vi "Get SQL formatted value.vi"(8 "error in (no error)":errorcluster, 11 "Column in":refnum<class "Ctrl Refnum Column.lvclass">) -> (0 "error out":errorcluster, 2 "Formatted Value":string, 3 "Column out":refnum<class "Ctrl Refnum Column.lvclass">)   [LabVIEW 2020, in "Basic Fields.lvlib" / "Ctrl Refnum Column.lvclass"]
uses:
  Ctrl Refnum Column.lvclass
  Ctrl Refnum Column.lvclass/Ctrl Refnum Column.ctl
  Basic Columns/Basic Columns/Column Class/Column Parent.lvclass
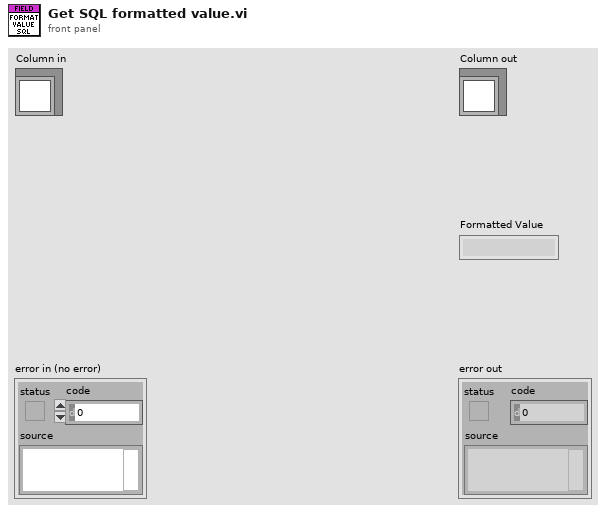
[diagram p1: front panel]
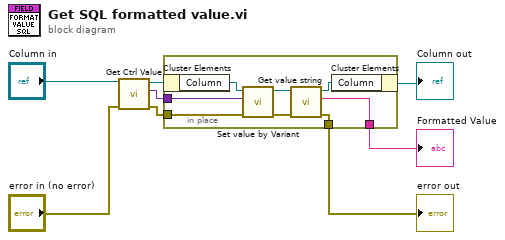
[diagram p0: block diagram]
diagram:
  n1 = call-dynamic "Get Ctrl Value.vi"("error in (no error)"="error in (no error)", "Ctrl Refnum Column in"="Column in") -> ("error out"=w3:errorcluster, "Ctrl Value"=w4:variant, "Ctrl Refnum Column out"=w6:refnum<class "Ctrl Refnum Column.lvclass">)  [unwired: 7 in]
  n2 = in-place {
    in-place-border: w4 -> [w15]
    in-place-border: w3 -> [w14]
    in-place-border: [w10] -> w2
    in-place-border: [w9] -> w1
    n3 = in-place-cluster #1(w6) -> ("Column"=w16:refnum<class "Column Parent.lvclass">)
    n4 = call-dynamic "Set value by Variant.vi"("error in (no error)"=w14, "Variant"=w15, "Column in"=w16) -> ("error out"=w12:errorcluster, "Column out"=w13:refnum<class "Column Parent.lvclass">)  [unwired: 7 in]
    n5 = call-dynamic "Get value string.vi"("error in (no error)"=w12, "Column in"=w13) -> ("error out"=w10:errorcluster, "Value"=w9:string, "Column out"=w11:refnum<class "Column Parent.lvclass">)  [unwired: 7 in]
    n6 = in-place-cluster #1("Column"=w11) -> (→"Column out":refnum<class "Ctrl Refnum Column.lvclass">)
  }
  "error out" <- w2
  "Formatted Value" <- w1
